vi "Read FrameTileCode.vi"(8 "error in (no error)":errorcluster, 11 "Menu in":refnum<class "Menu.lvclass">) -> (0 "error out":errorcluster, 2 "FrameTileCode":string, 3 "Menu out":refnum<class "Menu.lvclass">)   [LabVIEW 2019, in "RT_Game.lvlib" / "Menu.lvclass"]
uses:
  Menu.lvclass
  Menu.lvclass/Menu.ctl
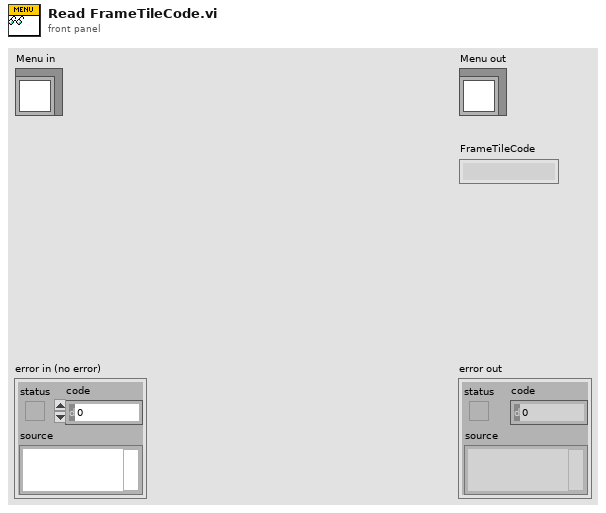
[diagram p1: front panel]
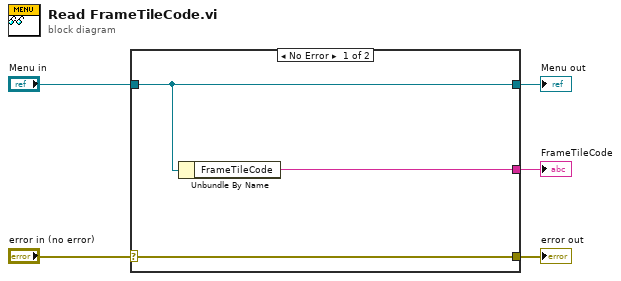
[diagram p0: block diagram]
diagram:
  n1 = case shown="No Error" "error in (no error)" {
    selector: "error in (no error)" -> [w8 w9]
    tunnel: [w8 w9] -> w4
    tunnel: [w7 w10] -> w2
    tunnel: "Menu in" -> [w7 w10]
    tunnel: [w6 _] -> w1
    frame No Error {
      n2 = Unbundle By Name(w7) -> ("FrameTileCode"=w6:string)
    }
    frame Error {
    }
  }
  "error out" <- w4
  "Menu out" <- w2
  "FrameTileCode" <- w1
